vi "List Waveforms.vi"(0 "VISA resource name":refnum<visa-resource-name>, 11 "error in (no error)":errorcluster) -> (4 "VISA resource name out":refnum<visa-resource-name>, 6 "Available Waveforms":string[](array[string]), 15 "error out":errorcluster)   [LabVIEW 2020, in "Agilent 681x Series.lvlib"]
doc: "Lists currently defined waveforms in the instrument storage.\n\n<B>Note:</B>\n\nThis VI lists the pre-defined waveforms <B>Sinusoid</B>, <B>Square</B> and <B>Clipped Sinusoid</B> as well."
uses:
  <instrlib>/Agilent 681x Series/Agilent 681x Series.lvlib
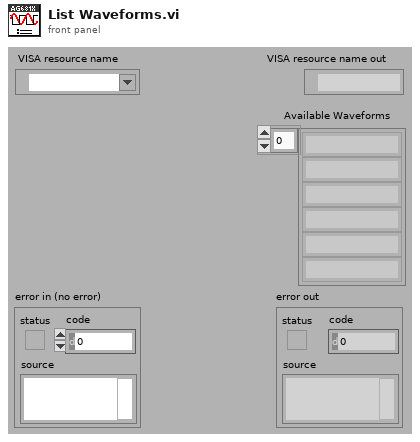
[diagram p1: front panel]
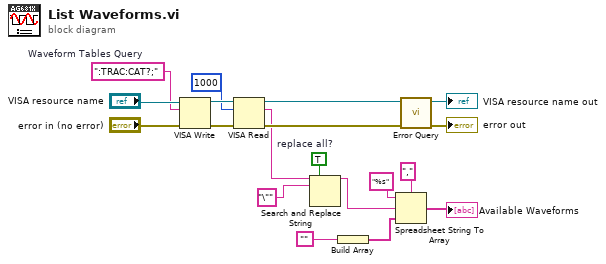
[diagram p0: block diagram]
diagram:
  w7 = TRUE  # replace all?
  w15 = ":TRAC:CAT?;"  # Waveform Tables Query
  n1 = VISA Write(VISA resource name="VISA resource name", write buffer=w15, error in (no error)="error in (no error)") -> (VISA resource name out=w14:refnum<visa-resource-name>, error out=w13:errorcluster)  [unwired: 1 out]
  n2 = VISA Read(VISA resource name=w14, byte count=u32 1000, error in (no error)=w13) -> (VISA resource name out=w12:refnum<visa-resource-name>, read buffer=w9:string, error out=w11:errorcluster)  [unwired: 1 out]
  n3 = Search and Replace String(replace all?=w7, input string=w9, search string="\"") -> (result string=w6:string)  [unwired: 5 in, 3 out]
  n4 = Build Array("") -> (w3:string[])
  n5 = Spreadsheet String To Array(delimiter (Tab)=",", format string="%s", spreadsheet string=w6, array type (2D Dbl)=w3) -> (array=→"Available Waveforms":string[])
  n6 = call <instrlib>:"Error Query.vi"("error in (no error)"=w11, "VISA resource name"=w12) -> ("error out"=→"error out":errorcluster, "VISA resource name out"=→"VISA resource name out":refnum<visa-resource-name>)  [unwired: 6 in, 2 out]
